vi "timeout.vi"(8 "error in (no error)":errorcluster, 11 "deviceHeartbeat in":refnum<class "deviceHeartbeat.lvclass">) -> (0 "error out":errorcluster, 2 "timeout?":bool, 3 "deviceHeartbeat out":refnum<class "deviceHeartbeat.lvclass">)   [LabVIEW 2016, in "deviceHeartbeat.lvclass"]
uses:
  deviceHeartbeat.lvclass
  deviceHeartbeat.lvclass/deviceHeartbeat.ctl
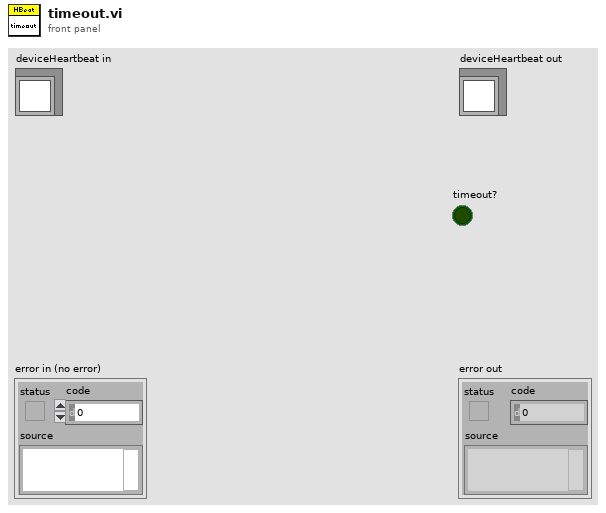
[diagram p1: front panel]
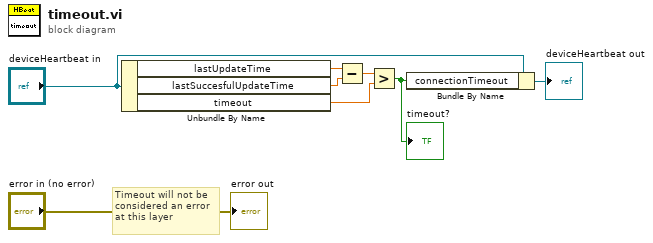
[diagram p0: block diagram]
diagram:
  # "Timeout will not be considered an error at this layer"
  n1 = Unbundle By Name("deviceHeartbeat in") -> ("lastUpdateTime"=w6:dbl, "lastSuccesfulUpdateTime"=w7:dbl, "timeout"=w5:dbl)
  n2 = Subtract(x=w6, y=w7) -> (x-y=w8:dbl)
  n3 = Greater?(x=w8, y=w5) -> (0:w1:bool)
  "timeout?" <- w1
  n4 = Bundle By Name(cluster="deviceHeartbeat in", "connectionTimeout"=w1) -> (→"deviceHeartbeat out":refnum<class "deviceHeartbeat.lvclass">)
  "error out" <- "error in (no error)"
